vi "X-A-SRC.vi"(8 "err in":errorcluster, 10 "src-nom":string) -> (0 "err out":errorcluster, 3 "SRC-X (s)":T1)   [LabVIEW 2010, in "lv_04.lvlib"]
uses:
  lv_04.lvlib
  commandes/cX.ctl
  commandes/cSTA_varid.ctl
  commandes/c_TDMS_ch_variable.ctl
  commandes/c_TDMS_ch_donnees.ctl
  commandes/c0-var-n.ctl
  commandes/cSTA_num_do_cr.ctl
  commandes/c02-do-num.ctl
  commandes/c04-stat-num.ctl
  commandes/cSTA_txt_do_cr.ctl
  commandes/c02-do-txt.ctl
  commandes/c04-stat-txt.ctl
  commandes/cSTA_dist.ctl
  commandes/c03-dist-S.ctl
  commandes/c0-dist-xy.ctl
  commandes/c03-dist-T.ctl
  commandes/c03-dist-SPC.ctl
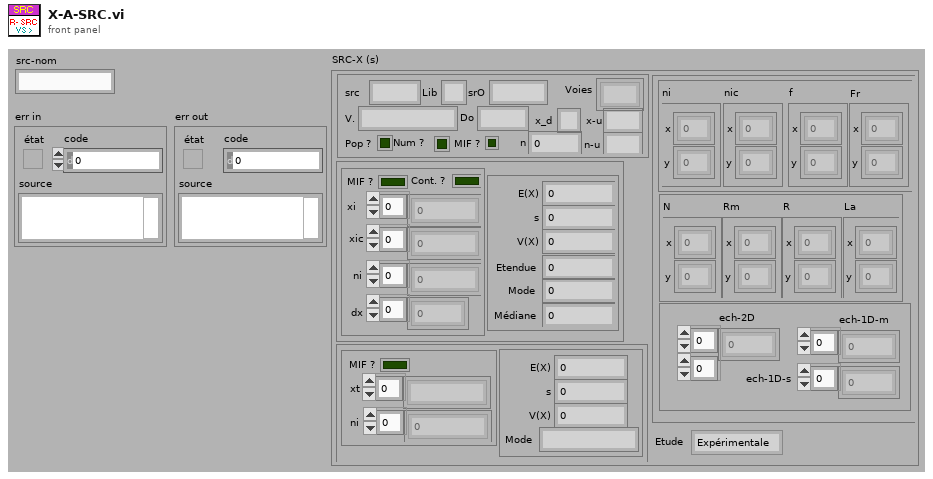
[diagram p1: front panel]
types:
  T1 = typedef "lv_04.lvlib/cX.ctl" = cluster{"src":T2, "num":T6, "txt":T9, "dist":T12, "Etude":enum16{"Expérimentale", "Modèle"}}
  T2 = typedef "lv_04.lvlib/cSTA_varid.ctl" = cluster{"src":string, "Lib":string, "srO":string, "V.":T3, "Voies":string[], "Do":T4, "n":T5, "Num ?":bool, "Pop ?":bool, "x_d":string, "x-u":string, "n-u":string, "MIF ?":bool}
  T3 = typedef "lv_04.lvlib/c_TDMS_ch_variable.ctl" = string
  T4 = typedef "lv_04.lvlib/c_TDMS_ch_donnees.ctl" = string
  T5 = typedef "lv_04.lvlib/c0-var-n.ctl" = i32
  T6 = typedef "lv_04.lvlib/cSTA_num_do_cr.ctl" = cluster{"do":T7, "sta":T8}
  T7 = typedef "lv_04.lvlib/c02-do-num.ctl" = cluster{"MIF ?":bool, "Cont. ?":bool, "xi":dbl[], "xic":dbl[], "ni":u32[], "dx":dbl[]}
  T8 = typedef "lv_04.lvlib/c04-stat-num.ctl" = cluster{"E(X)":dbl, "s":dbl, "V(X) ":dbl, "Etendue":dbl, "Mode":dbl, "Médiane":dbl}
  T9 = typedef "lv_04.lvlib/cSTA_txt_do_cr.ctl" = cluster{"do":T10, "sta":T11}
  T10 = typedef "lv_04.lvlib/c02-do-txt.ctl" = cluster{"xt":string[], "ni":dbl[], "MIF ?":bool}
  T11 = typedef "lv_04.lvlib/c04-stat-txt.ctl" = cluster{"E(X)":dbl, "s":dbl, "V(X) ":dbl, "Mode":string}
  T12 = typedef "lv_04.lvlib/cSTA_dist.ctl" = cluster{"S":T13, "T":T15, "spc":T16}
  T13 = typedef "lv_04.lvlib/c03-dist-S.ctl" = cluster{"nic":T14, "f":T14, "Fr":T14, "ni":T14}
  T14 = typedef "lv_04.lvlib/c0-dist-xy.ctl" = cluster{"x":dbl[], "y":dbl[]}
  T15 = typedef "lv_04.lvlib/c03-dist-T.ctl" = cluster{"N":T14, "Rm":T14, "R":T14, "La":T14}
  T16 = typedef "lv_04.lvlib/c03-dist-SPC.ctl" = cluster{"ech-2D":dbl[][], "ech-1D-m":dbl[], "ech-1D-s":dbl[]}
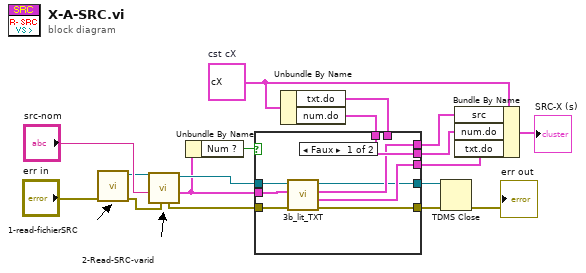
[diagram p0: block diagram]
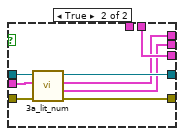
[diagram p2: hidden frame]
diagram:
  w3 = T1 {"src"={"src"="", "Lib"="", "srO"="", "V."="", "Voies"=[], "Do"="", "n"=0, "Num ?"=FALSE, "Pop ?"=FALSE, "x_d"="", "x-u"="", "n-u"="", "MIF ?"=FALSE}, "num"={"do"={"MIF ?"=FALSE, "Cont. ?"=FALSE, "xi"=[], "xic"=[], "ni"=[], "dx"=[]}, "sta"={"E(X)"=0.0, "s"=0.0, "V(X) "=0.0, "Etendue"=0.0, "Mode"=0.0, "Médiane"=0.0}}, "txt"={"do"={"xt"=[], "ni"=[], "MIF ?"=FALSE}, "sta"={"E(X)"=0.0, "s"=0.0, "V(X) "=0.0, "Mode"=""}}, "dist"={"S"={"nic"={"x"=[], "y"=[]}, "f"={"x"=[], "y"=[]}, "Fr"={"x"=[], "y"=[]}, "ni"={"x"=[], "y"=[]}}, "T"={"N"={"x"=[], "y"=[]}, "Rm"={"x"=[], "y"=[]}, "R"={"x"=[], "y"=[]}, "La"={"x"=[], "y"=[]}}, "spc"={"ech-2D"=[], "ech-1D-m"=[], "ech-1D-s"=[]}}, "Etude"=enum."Expérimentale"}  # cst cX
  n1 = call "1-read-fichierSRC.vi"("err in"="err in") -> ("err out"=w17:errorcluster, "tdms file out"=w16:refnum<k34>)  [unwired: 4 in, 1 out]
  n2 = call "2-Read-SRC-varid.vi"("err in"=w17, "code src"="src-nom", "tdms in"=w16) -> ("varid"=w11:T2, "tdms out"=w13:refnum<k34>, "error out"=w12:errorcluster)  [unwired: 4 in, 2 out]
  n3 = Unbundle By Name(w11) -> ("Num ?"=w9:bool)
  n4 = Unbundle By Name(w3) -> ("txt.do"=w1:T10, "num.do"=w2:T7)
  n5 = case shown="Faux" w9 {
    tunnel: w13 -> [w25 w33]
    tunnel: w12 -> [w23 w31]
    tunnel: w11 -> [w24 w32]
    tunnel: [w19 w30] -> w6
    tunnel: [w20 w29] -> w10
    tunnel: [w26 w28] -> w8
    tunnel: [w22 w27] -> w5
    tunnel: [w21 w34] -> w7
    tunnel: w2 -> [w26 _]
    tunnel: w1 -> [_ w34]
    frame False {
      n6 = call "3b_lit_TXT.vi"("err in"=w23, "src"=w24, "tdms in"=w25) -> ("err out"=w22:errorcluster, "do_txt"=w21:T10, "src"=w20:T2, "tdms out"=w19:refnum<k34>)  [unwired: 1 in]
    }
    frame True {
      n7 = call "3a_lit_num.vi"("erreur in"=w31, "varid"=w32, "tdms file in"=w33) -> ("error out"=w27:errorcluster, "do_num"=w28:T7, "varid"=w29:T2, "tdms file out"=w30:refnum<k34>)  [unwired: 1 in]
    }
  }
  n8 = TDMS Close(8:w5, 11:w6) -> (0:→"err out":errorcluster)  [unwired: 1 out]
  n9 = Bundle By Name(cluster=w3, "src"=w10, "num.do"=w8, "txt.do"=w7) -> (→"SRC-X (s)":T1)
